vi "ATMonochromator_getEvent_wavelength.vi"(8 "error in (no error)":errorcluster, 11 "logevent_wavelength_Ctl":T1) -> (0 "error out":errorcluster, 2 "function return":i32, 3 "logevent_wavelength_Ctl out":T1)   [LabVIEW 2016, in "SALLV_ATMonochromator.lvlib"]
doc: "int ATMonochromator_shm_getEvent_wavelengthLV(ATMonochromator_logevent_wavelengthLV *logevent_wavelength_Ctl );"
uses:
  SALLV_ATMonochromator.lvlib
  DataTypes/logevent_wavelength.ctl
  SALLV_ATMonochromator.so
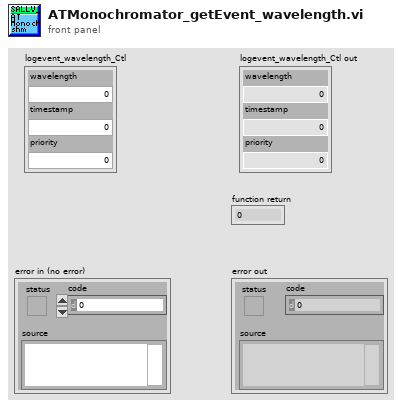
[diagram p1: front panel]
types:
  T1 = typedef "SALLV_ATMonochromator.lvlib/logevent_wavelength.ctl" = cluster{"wavelength":sgl, "timestamp":dbl, "priority":i32}
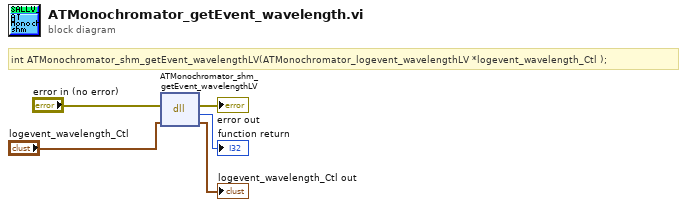
[diagram p0: block diagram]
diagram:
  # "int ATMonochromator_shm_getEvent_wavelengthLV(ATMonochromator_logevent_wavelengthLV *logevent_wavelength_Ctl );"
  n1 = dll-call lib="home/harini/tcs/SALLV_ATMonochromator/SALLV_ATMonochromator.*" fn="ATMonochromator_shm_getEvent_wavelengthLV"(error in="error in (no error)", "logevent_wavelength_Ctl"="logevent_wavelength_Ctl") -> (error out=→"error out":errorcluster, →"function return":i32, "logevent_wavelength_Ctl"=→"logevent_wavelength_Ctl out":T1)  [unwired: 2 in, 1 out]
